vi "Convert to String.vi"(8 "error in (no error)":errorcluster, 10 "data":variant) -> (0 "error out":errorcluster, 2 "String":string)   [LabVIEW 2023, in "uData.lvlib" / "uData.lvclass"]
doc: "Convert incoming data type to string."
uses:
  uData.lvclass
  uConvertible.lvclass
  uData.lvclass/uData.ctl
  Accessor - Set.vi
  Inline Write.vi
  Condition Tag Names.vi
  Condition Tag Name.vi
  Blank Key Reserved String.vi
  <vilib>/Utility/error.llb/Error Cluster From Error Code.vi
  Breakdown Cluster.vi
  <vilib>/ErrorRing/Error Ring.xnode
  <vilib>/Utility/Data Type/NI_Data Type.lvlib
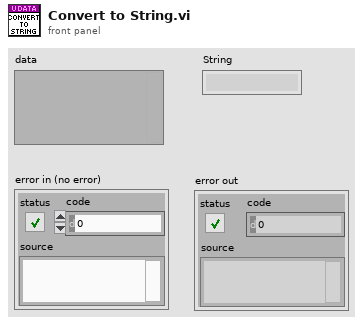
[diagram p1: front panel]
types:
  T1 = typedef "NI_Data Type.lvlib/Data Type.ctl" = enum8{"Invalid Type", "Void", "I8", "I16", "I32", "I64", "U8", "U16", "U32", "U64", "Single Float", "Double Float", "Extended Float", "Single Complex", "Double Complex", "Extended Complex", "Enum U8", "Enum U16", "Enum U32", "Enum U64", "Single Float With Unit", "Double Float With Unit", "Extended Float With Unit", "Single Complex with Unit", "Double Complex with Unit", "Extended Complex with Unit", "Boolean", "String", "Path", "Picture", "Tag", "Array", "Cluster", "Variant", "LV Variant", "Waveform", "Timestamp", "Digital Waveform", "Digital Data", "ExpressData", "Refnum", "External Data", "VI", "Poly VI", "LabVIEW Class Instance", "Fixed Point", "Set Collection", "Map Collection"}
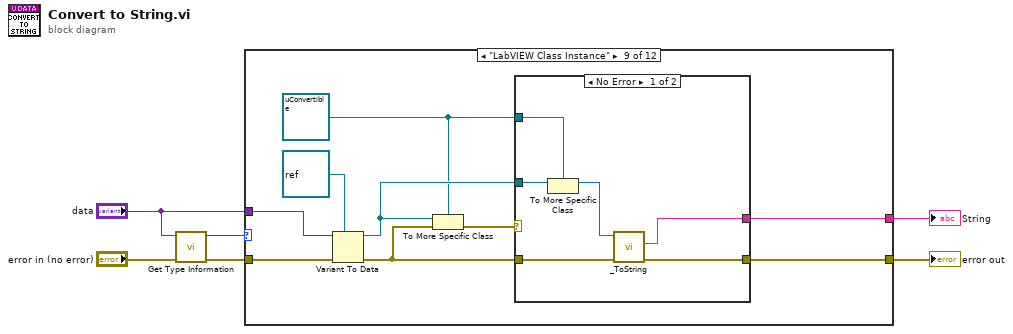
[diagram p0: block diagram]
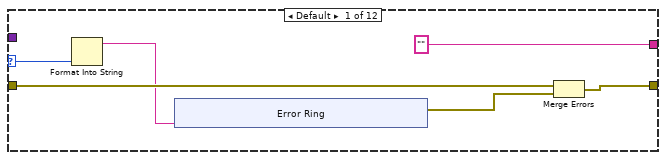
[diagram p2: hidden frame]
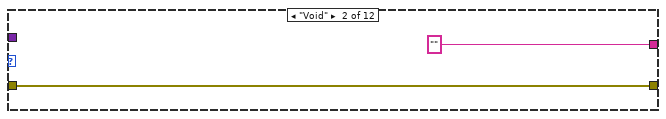
[diagram p3: hidden frame]
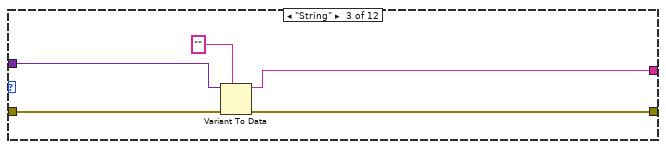
[diagram p4: hidden frame]
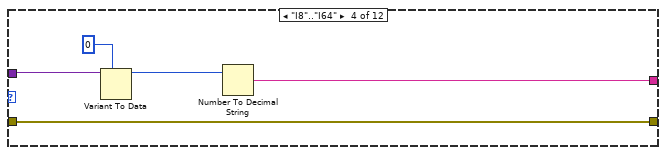
[diagram p5: hidden frame]
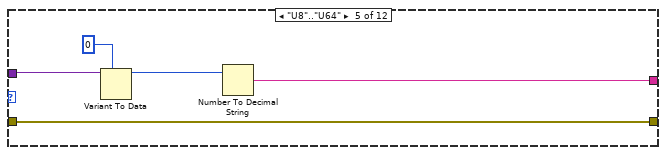
[diagram p6: hidden frame]
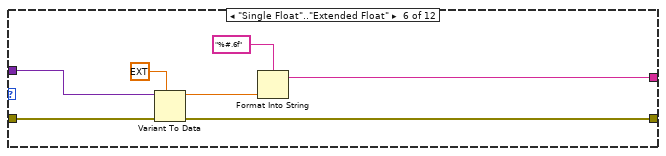
[diagram p7: hidden frame]
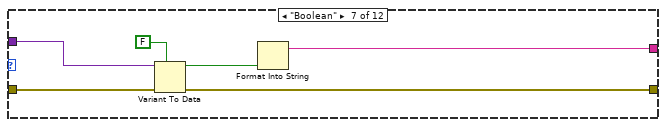
[diagram p8: hidden frame]
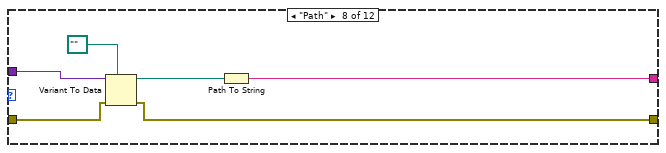
[diagram p9: hidden frame]
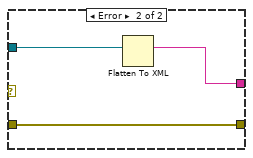
[diagram p10: hidden frame]
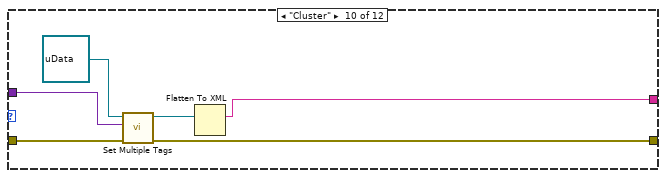
[diagram p11: hidden frame]
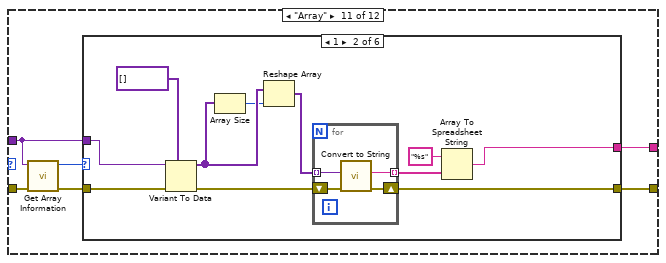
[diagram p12: hidden frame]
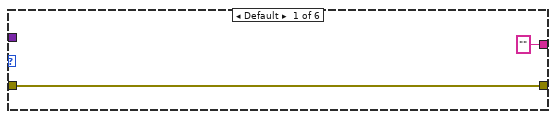
[diagram p13: hidden frame]
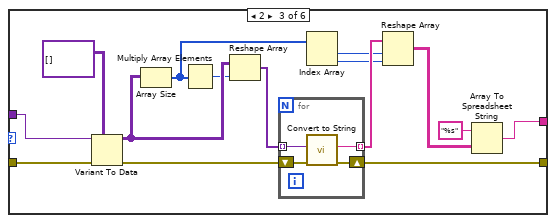
[diagram p14: hidden frame]
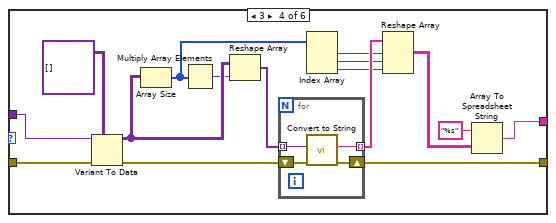
[diagram p15: hidden frame]
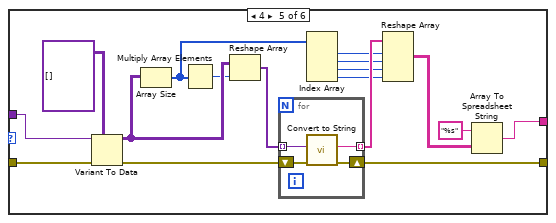
[diagram p16: hidden frame]
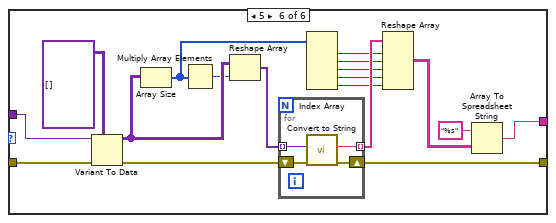
[diagram p17: hidden frame]
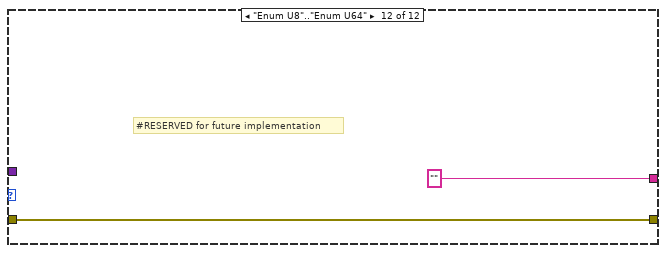
[diagram p18: hidden frame]
diagram:
  n1 = call <vilib>:"Get Type Information.vi"("error in (no error)"="error in (no error)", "variant"="data") -> ("error out"=w3:errorcluster, "type"=w5:T1)  [unwired: 5 in, 3 out]
  n2 = case shown="\"LabVIEW Class Instance\"" w5 {
    selector: w5 -> [w11 _ _ _ _ _ _ _ _ _ _ _]
    tunnel: [w7 w20 w25 w30 w35 w42 w48 w52 w57 w76 w80 w186] -> w4
    tunnel: w3 -> [w12 w20 w26 w30 w35 w41 w47 w53 w64 w79 w85 w186]
    tunnel: ["" "" w23 w31 w36 w43 w49 w54 w60 w74 w81 "" ("xml string")] -> w2
    tunnel: "data" -> [_ _ w24 w29 w34 w40 w46 w55 w63 w78 w82 _]
    frame Default {
      n3 = Format Into String(w11) -> (resulting string=w10:string)  [unwired: 3 in, 1 out]
      n4 = xnode "Error Ring"("parameter 0"=w10) -> ("error out"=w8:errorcluster)
      n5 = Merge Errors(w12, w8) -> (w7:errorcluster)
    }
    frame "Void" {
    }
    frame "String" {
      n6 = Variant To Data(error in=w26, type="", Variant=w24) -> (data=w23:string, error out=w25:errorcluster)
    }
    frame "I8".."I64" {
      n7 = Variant To Data(type=i64 0, Variant=w29) -> (data=w28:i64)  [unwired: 1 in, 1 out]
      n8 = Number To Decimal String(number=w28) -> (decimal integer string=w31:string)  [unwired: 1 in]
    }
    frame "U8".."U64" {
      n9 = Variant To Data(type=u64 0, Variant=w34) -> (data=w33:u64)  [unwired: 1 in, 1 out]
      n10 = Number To Decimal String(number=w33) -> (decimal integer string=w36:string)  [unwired: 1 in]
    }
    frame "Single Float".."Extended Float" {
      n11 = Variant To Data(error in=w41, type=ext 0.0, Variant=w40) -> (data=w39:ext, error out=w42:errorcluster)
      n12 = Format Into String(format string="%#.6f", w39) -> (resulting string=w43:string)  [unwired: 2 in, 1 out]
    }
    frame "Boolean" {
      n13 = Variant To Data(error in=w47, type=FALSE, Variant=w46) -> (data=w45:bool, error out=w48:errorcluster)
      n14 = Format Into String(w45) -> (resulting string=w49:string)  [unwired: 3 in, 1 out]
    }
    frame "Path" {
      n15 = Variant To Data(error in=w53, type=path "", Variant=w55) -> (data=w50:path, error out=w52:errorcluster)
      n16 = Path To String(path=w50) -> (string=w54:string)
    }
    frame "LabVIEW Class Instance" {
      w56 = refnum<class "uConvertible.lvclass"> refnum ("uData.lvlib:uConvertible.lvclass")
      n17 = Variant To Data(error in=w64, type=refnum<class> refnum ("LabVIEW Object"), Variant=w63) -> (data=w59:refnum<class>, error out=w58:errorcluster)
      n18 = To More Specific Class(target class=w56, reference=w59, error in=w58) -> (error out=w61:errorcluster)  [unwired: 1 out]
      n19 = case shown="No Error" w61 {
        tunnel: [w68 w73] -> w60
        tunnel: w59 -> [w67 w72]
        tunnel: w58 -> [w69 w71]
        tunnel: [w70 w71] -> w57
        tunnel: w56 -> [w66 _]
        frame No Error {
          n20 = To More Specific Class(target class=w66, reference=w67) -> (specific class reference=w65:refnum<class "uConvertible.lvclass">)  [unwired: 1 in, 1 out]
          n21 = call-dynamic "_ToString.vi"("error in (no error)"=w69, "uConvertible in"=w65) -> ("error out"=w70:errorcluster, "ToString"=w68:string)  [unwired: 7 in, 1 out]
        }
        frame Error {
          n22 = Flatten To XML(6:w72) -> (2:w73:string)
        }
      }
    }
    frame "Cluster" {
      n23 = call "Set Multiple Tags.vi"("error in (no error)"=w79, "Cluster"=w78, "uData in"=refnum<class "uData.lvclass"> refnum ("iData in")) -> ("error out"=w76:errorcluster, "uData out"=w75:refnum<class "uData.lvclass">)  [unwired: 5 in, 2 out]
      n24 = Flatten To XML(6:w75) -> (2:w74:string)
    }
    frame "Array" {
      n25 = call <vilib>:"Get Array Information.vi"("error in (no error)"=w85, "variant"=w82) -> ("error out"=w84:errorcluster, "number of dimensions"=w83:i32)  [unwired: 6 in, 2 out]
      n26 = case shown="1" w83 {
        tunnel: w84 -> [w87 w98 w117 w137 w158 w180]
        tunnel: [w87 w91 w111 w131 w152 w174] -> w80
        tunnel: w82 -> [_ w96 w115 w135 w156 w178]
        tunnel: ["" ("spreadsheet string") w88 w109 w129 w150 w172] -> w81
        frame Default {
        }
        frame 1 {
          n27 = Variant To Data(error in=w98, type=variant[] [], Variant=w96) -> (data=w95:variant[], error out=w92:errorcluster)
          n28 = Array Size(array=w95) -> (size(s)=w94:i32)
          n29 = Reshape Array(w95, w94) -> (w93:variant[])
          n30 = for {
            shift-right: [w101] -> w91
            shift-left: w92 -> [w102]
            tunnel: w93 -> [w100] mode=indexing
            tunnel: [w99] -> w90 mode=indexing
            n31 = call "Convert to String.vi"("error in (no error)"=w102, "data"=w100) -> ("error out"=w101:errorcluster, "String"=w99:string)  [unwired: 8 in]
          }
          n32 = Array To Spreadsheet String(array=w90, 3:"%s" ("format string")) -> (spreadsheet string=w88:string)  [unwired: 1 in]
        }
        frame 2 {
          n33 = Variant To Data(error in=w117, type=variant[][] [], Variant=w115) -> (data=w114:variant[][], error out=w112:errorcluster)
          n34 = Array Size(array=w114) -> (size(s)=w106:i32[])
          n35 = Multiply Array Elements(1:w106) -> (0:w108:i32)
          n36 = Reshape Array(w114, w108) -> (w113:variant[])
          n37 = for {
            shift-right: [w120] -> w111
            shift-left: w112 -> [w121]
            tunnel: w113 -> [w119] mode=indexing
            tunnel: [w118] -> w107 mode=indexing
            n38 = call "Convert to String.vi"("error in (no error)"=w121, "data"=w119) -> ("error out"=w120:errorcluster, "String"=w118:string)  [unwired: 8 in]
          }
          n39 = Index Array(array=w106) -> (element #1=w105:i32, element #2=w104:i32)  [unwired: 2 in]
          n40 = Reshape Array(w107, w105, w104) -> (w103:string[][])
          n41 = Array To Spreadsheet String(array=w103, 3:"%s" ("format string")) -> (spreadsheet string=w109:string)  [unwired: 1 in]
        }
        frame 3 {
          n42 = Variant To Data(error in=w137, type=variant[][][] [], Variant=w135) -> (data=w134:variant[][][], error out=w132:errorcluster)
          n43 = Array Size(array=w134) -> (size(s)=w126:i32[])
          n44 = Multiply Array Elements(1:w126) -> (0:w128:i32)
          n45 = Reshape Array(w134, w128) -> (w133:variant[])
          n46 = for {
            shift-right: [w140] -> w131
            shift-left: w132 -> [w141]
            tunnel: w133 -> [w139] mode=indexing
            tunnel: [w138] -> w127 mode=indexing
            n47 = call "Convert to String.vi"("error in (no error)"=w141, "data"=w139) -> ("error out"=w140:errorcluster, "String"=w138:string)  [unwired: 8 in]
          }
          n48 = Index Array(array=w126) -> (element #1=w125:i32, element #2=w124:i32, element #3=w122:i32)  [unwired: 3 in]
          n49 = Reshape Array(w127, w125, w124, w122) -> (w123:string[][][])
          n50 = Array To Spreadsheet String(array=w123, 3:"%s" ("format string")) -> (spreadsheet string=w129:string)  [unwired: 1 in]
        }
        frame 4 {
          n51 = Variant To Data(error in=w158, type=variant[][][][] [], Variant=w156) -> (data=w155:variant[][][][], error out=w153:errorcluster)
          n52 = Array Size(array=w155) -> (size(s)=w147:i32[])
          n53 = Multiply Array Elements(1:w147) -> (0:w149:i32)
          n54 = Reshape Array(w155, w149) -> (w154:variant[])
          n55 = for {
            shift-right: [w161] -> w152
            shift-left: w153 -> [w162]
            tunnel: w154 -> [w160] mode=indexing
            tunnel: [w159] -> w148 mode=indexing
            n56 = call "Convert to String.vi"("error in (no error)"=w162, "data"=w160) -> ("error out"=w161:errorcluster, "String"=w159:string)  [unwired: 8 in]
          }
          n57 = Index Array(array=w147) -> (element #1=w146:i32, element #2=w145:i32, element #3=w143:i32, element #4=w142:i32)  [unwired: 4 in]
          n58 = Reshape Array(w148, w146, w145, w143, w142) -> (w144:string[][][][])
          n59 = Array To Spreadsheet String(array=w144, 3:"%s" ("format string")) -> (spreadsheet string=w150:string)  [unwired: 1 in]
        }
        frame 5 {
          n60 = Variant To Data(error in=w180, type=variant[][][][][] [], Variant=w178) -> (data=w177:variant[][][][][], error out=w175:errorcluster)
          n61 = Array Size(array=w177) -> (size(s)=w169:i32[])
          n62 = Multiply Array Elements(1:w169) -> (0:w171:i32)
          n63 = Reshape Array(w177, w171) -> (w176:variant[])
          n64 = for {
            shift-right: [w183] -> w174
            shift-left: w175 -> [w184]
            tunnel: w176 -> [w182] mode=indexing
            tunnel: [w181] -> w170 mode=indexing
            n65 = call "Convert to String.vi"("error in (no error)"=w184, "data"=w182) -> ("error out"=w183:errorcluster, "String"=w181:string)  [unwired: 8 in]
          }
          n66 = Index Array(array=w169) -> (element #1=w168:i32, element #2=w167:i32, element #3=w165:i32, element #4=w164:i32, element #5=w163:i32)  [unwired: 5 in]
          n67 = Reshape Array(w170, w168, w167, w165, w164, w163) -> (w166:string[][][][][])
          n68 = Array To Spreadsheet String(array=w166, 3:"%s" ("format string")) -> (spreadsheet string=w172:string)  [unwired: 1 in]
        }
      }
    }
    frame "Enum U8".."Enum U64" {
      # "#RESERVED for future implementation"
    }
  }
  "String" <- w2
  "error out" <- w4
